vi "Package.vi"   [LabVIEW 2018, in "Scripts.lvlib"]
doc: "Builds a VI package (vip) for this project for LabVIEW 2009."
uses:
  Scripts.lvlib
  <vilib>/Field R&D Services/Labricator/Toolkit/Controls/LabVIEW Versions.ctl
  <vilib>/Field R&D Services/Labricator/Toolkit/Labricator.lvlib
panel:
  # "Overview: Builds a VI Package (vip) for LabVIEW versions >= 2014\nRequirements: LabVIEW 2014, VIPM Pro, VIPM API, Application Builder\nInstructions: Run this VI.\n\nThis VI attempts automate the building the VIP file for this add-on as much as possible. If VIPM Pro is not available, then the VIPM API will not work, and the building of the package must be done manually. This VI automates the following manual steps:\n\n1. Save the current project for LabVIEW 2014\n    a. From the Project Explorer window, select File>>Save for Previous Version... A new dialog will appear.\n    b. Select 14.0 from the drop down menu.\n    c. Click Save.... A new dialog will appear. Create a \"<project root>\\target\\14.0\" folder hierarchy in the root project folder (same location as the \n        project file, .lvproj) if it does not already exist.\n    d. Click OK. All of the contents of the project will be saved to LabVIEW 2014.\n2. Copy the Help source to the target output\n    a. Start Windows Explorer.\n    b. Navigate to the \"<project root>\\src\" folder in Windows Explorer.\n    c. Copy the \"Help\" folder to the \"<project root>\\target\\14.0\\src\" location.\n3. Start LabVIEW 2014 and open the \"<project root>\\target\\14.0\\Labstache.lvproj\" file created in Step 1. Do NOT open any file in \n    the \"<project root>\\target\\14.0\" folder in any other version of LabVIEW.\n4. Open each Source Distribution build specification under the \"Build Specifications\" tree item in the Project Explorer and change the Output  \n    Destination to \"<project root?\\target\\14.0\\builds\". Save and close each build specification. \n5. Build all Source Distributions defined under \"Build Specifications\" tree item in the Project Explorer. A new \"<project root>\\target\\14.0\\builds\" \n    folder will be created with a sub-folder for each component.\n6. Expand the Configurations virtual folder in the Project Explorer and double click on the \"Labstache.vipb\" file. This will start the VIPM \n    application.\n7. Click the \"Build\" icon near the top of the window for the package specification. Do NOT alter any values, but ensure \"2014\" is selected at the top \n    right.\n8. Once the package is built, it will be available at \"<project root>\\target\\14.0\\packages\". \n\nNote, any version newer than LabVIEW 2014 can be used to run this VI and still have the package built for LabVIEW 2014, but the LabVIEW 2014 development environment must be installed.\n\nWhen this VI runs, it will automatically start LabVIEW 2014, build all of the components, start VIPM, build the package, then close both LabVIEW 2014 and VIPM. Another VI, \"Build Target.vi\" will run during this process. Do not abort or close the VI will running. LabVIEW 2014 cannot be running before this VI runs."
types:
  T1 = typedef "Labricator.lvlib/LabVIEW Versions.ctl" = enum16{"2009", "2010", "2011", "2012", "2013", "2014", "2015", "2016", "2017", "2018"}
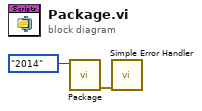
[diagram p0: block diagram]
diagram:
  n1 = call <vilib>:"Package.vi"("LabVIEW Previous Version"=LabVIEW_Versions."2014") -> ("Error Out"=w2:errorcluster)  [unwired: 10 in]
  n2 = call <vilib>:"Simple Error Handler.vi"("error in (no error)"=w2) -> ()  [unwired: 4 in, 5 out]
